vi "Set VI Inlining.vi"(8 "error in (no error)":errorcluster, 10 "Inline VI":bool, 11 "vi ref in":refnum<vi>) -> (0 "error out":errorcluster, 3 "vi ref out":refnum<vi>)   [LabVIEW 2020, in "Build Automation.lvlib"]
uses:
  Build Automation.lvlib
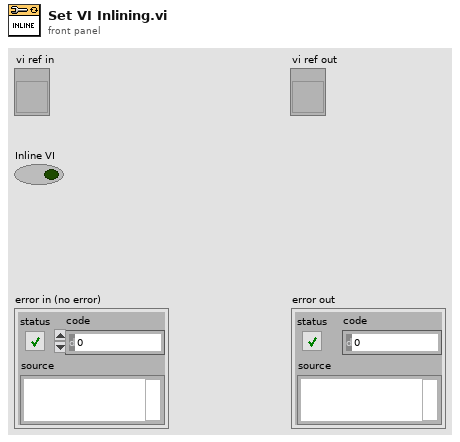
[diagram p1: front panel]
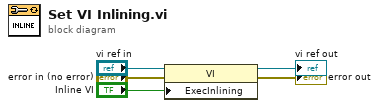
[diagram p0: block diagram]
diagram:
  n1 = property class="VI"(reference="vi ref in", error in="error in (no error)", "ExecInlining"="Inline VI") -> (reference out=→"vi ref out":refnum<vi>, error out=→"error out":errorcluster)
